vi "BASE.SaveConfig.vi"(8 "error in (no error)":errorcluster, 10 "config file path":path, 11 "BASE.Device in":refnum<class "BASE.Device.lvclass">) -> (0 "error out":errorcluster, 3 "BASE.Device out":refnum<class "BASE.Device.lvclass">)   [LabVIEW 2019, in "BASE.Device.lvlib" / "BASE.Device.lvclass"]
uses:
  BASE.Device.lvclass
  BASE.Device.lvclass/BASE.Device.ctl
  BASE/BASE/BASE.lvclass
  <vilib>/Utility/config.llb/NI_LVConfig.lvlib
panel:
  out "class name":string
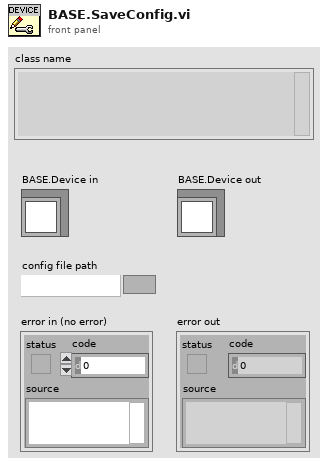
[diagram p1: front panel]
types:
  T1 = typedef "BASE.Device.lvlib/BASE.Device.lvclass/config--cluster.ctl" = cluster{"Connect Timeout":i32, "Check Timeout":i32, "Read Timeout":i32}
  T2 = typedef "NI_LVConfig.lvlib/Config Data RefNum.ctl" = refnum<k1>
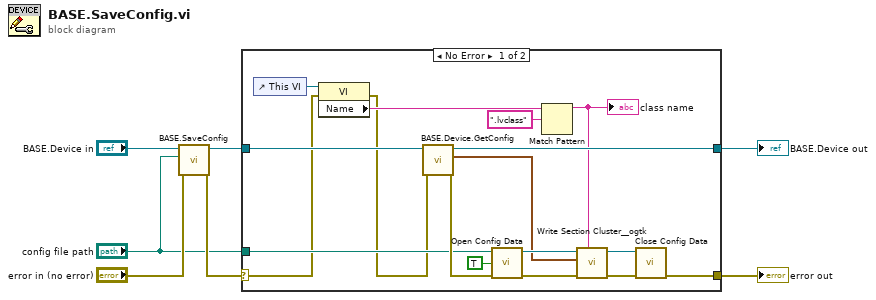
[diagram p0: block diagram]
diagram:
  n1 = call-parent "BASE.SaveConfig.vi"("error in (no error)"="error in (no error)", "config file path"="config file path", "BASE in"="BASE.Device in") -> ("error out"=w4:errorcluster, "BASE out"=w5:refnum<class "BASE.Device.lvclass">)  [unwired: 7 in]
  n2 = case shown="No Error" w4 {
    selector: w4 -> [w13 w26]
    tunnel: [w18 w26] -> w2
    tunnel: [w16 w25] -> w3
    tunnel: w5 -> [w15 w25]
    tunnel: "config file path" -> [w17 _]
    frame No Error {
      n3 = control-ref of="This VI"() -> (w14:refnum<vi>)
      n4 = property class="VI"(reference=w14, error in=w13) -> (error out=w9:errorcluster, "Name"=w12:string)  [unwired: 1 out]
      n5 = call "BASE.Device.GetConfig.vi"("error in (no error)"=w9, "BASE.Device in"=w15) -> ("error out"=w19:errorcluster, "config"=w23:T1, "BASE.Device out"=w16:refnum<class "BASE.Device.lvclass">)  [unwired: 7 in]
      n6 = call <vilib>:"Open Config Data.vi"("error in (no error)"=w19, "create file if necessary (T)"=TRUE, "configuration file path"=w17) -> ("error out"=w22:errorcluster, "refnum"=w24:T2)  [unwired: 6 in, 1 out]
      n7 = Match Pattern(string=w12, regular expression=".lvclass") -> (before substring=w10:string)  [unwired: 1 in, 3 out]
      "class name" <- w10
      n8 = call <userlib>:"Write Section Cluster__ogtk.vi"("section (optional)"=w10, "error in (no error)"=w22, "Section Formatted Cluster"=w23, "refnum"=w24) -> ("error out"=w21:errorcluster, "dup refnum"=w20:T2)  [unwired: 6 in]
      n9 = call <vilib>:"Close Config Data.vi"("error in (no error)"=w21, "refnum"=w20) -> ("error out"=w18:errorcluster)  [unwired: 8 in, 1 out]
    }
    frame Error {
    }
  }
  "error out" <- w2
  "BASE.Device out" <- w3
